vi "Enum to Boolean Number.vi"(4 "Button Selection":T1[](array[typedef])=[enum."A"]) -> (0 "number":u32)   [LabVIEW 2018]
uses:
  Buttons.ctl
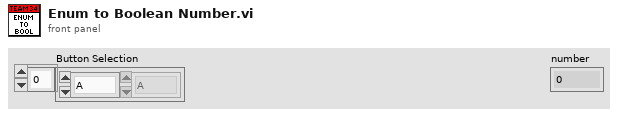
[diagram p1: front panel]
types:
  T1 = typedef "Buttons.ctl" = enum16{"A", "B", "X", "Y", "LB", "RB", "Back", "Start", "LS", "RS"}
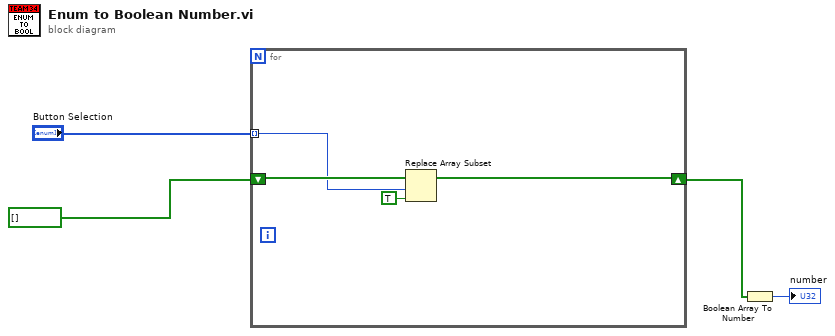
[diagram p0: block diagram]
diagram:
  n1 = for {
    tunnel: "Button Selection" -> [w7] mode=indexing
    shift-right: [w5] -> w2
    shift-left: bool[] [] -> [w8]
    n2 = Replace Array Subset(array=w8, new element=TRUE ("new element/subarray"), index=w7) -> (w5:bool[])
  }
  n3 = Boolean Array To Number(Boolean array=w2) -> (number=→"number":u32)
